vi "Update UI.vi"(8 "error in (no error)":errorcluster, 11 "Editor.lvclass in":refnum<data-value>) -> (0 "error out":errorcluster, 3 "Editor.lvclass out":refnum<data-value>)   [LabVIEW 2015, in "Editor.lvclass"]
uses:
  Editor.lvclass
  Project.lvclass
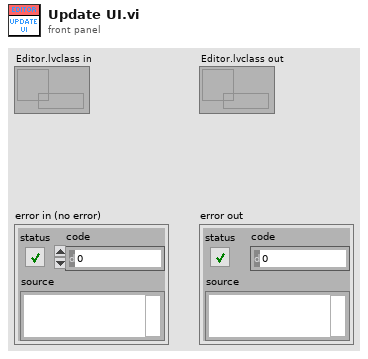
[diagram p1: front panel]
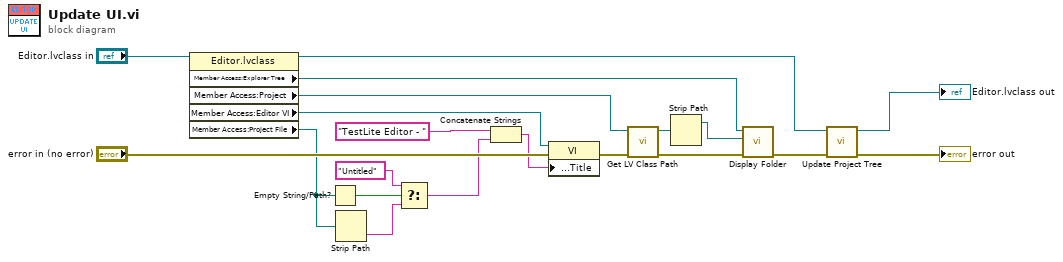
[diagram p0: block diagram]
diagram:
  n1 = property class="Editor.lvclass"(reference="Editor.lvclass in") -> (reference out=w19:refnum<data-value>, "Member Access:Explorer Tree"=w11:refnum<vi>, "Member Access:Project"=w12:refnum<class "Project.lvclass">, "Member Access:Editor VI"=w10:refnum<vi>, "Member Access:Project File"=w7:path)  [unwired: 1 in, 1 out]
  n2 = Empty String/Path?(string/path=w7) -> (empty?=w6:bool)
  n3 = Strip Path(path=w7) -> (name=w5:string)  [unwired: 1 out]
  n4 = Select(t="Untitled", s=w6, f=w5) -> (s? t:f=w2:string)
  n5 = Concatenate Strings("TestLite Editor - ", w2) -> (w1:string)
  n6 = property class="VI"(reference=w10, error in="error in (no error)", "Front Panel.Title"=w1) -> (error out=w8:errorcluster)  [unwired: 1 out]
  n7 = call <vilib>:"Get LV Class Path.vi"("error in (no error)"=w8, "object"=w12) -> ("error out"=w15:errorcluster, "class path"=w16:path)  [unwired: 8 in]
  n8 = Strip Path(path=w16) -> (stripped path=w17:path)  [unwired: 1 out]
  n9 = call "Display Folder.vi"("error in (no error)"=w15, "Folder in"=w17, "TreeControl in"=w11) -> ("error out"=w14:errorcluster)  [unwired: 6 in, 2 out]
  n10 = call "Update Project Tree.vi"("error in (no error)"=w14, "Editor.lvclass in"=w19) -> ("error out"=→"error out":errorcluster, "Editor.lvclass out"=→"Editor.lvclass out":refnum<data-value>)  [unwired: 8 in]
